vi "WPS_comm.vi"(0 "Path to Batch":string, 1 "Path to Exe":string, 2 "WPS IP:Port":string, 3 "Username":string, 4 "Password":string, 5 "Command":string) -> (14 "standard output":string, 15 "standard error":string, 16 "return code":i32, 19 "error out":errorcluster)   [LabVIEW 2016]
panel:
  out "Time (ms)":u32
  out "Complete command":string
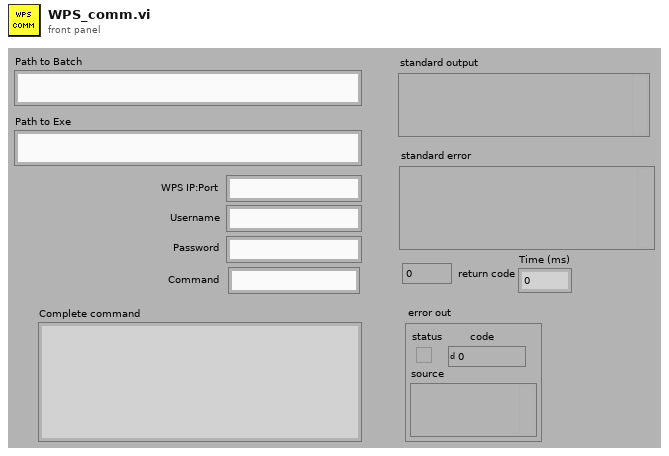
[diagram p1: front panel]
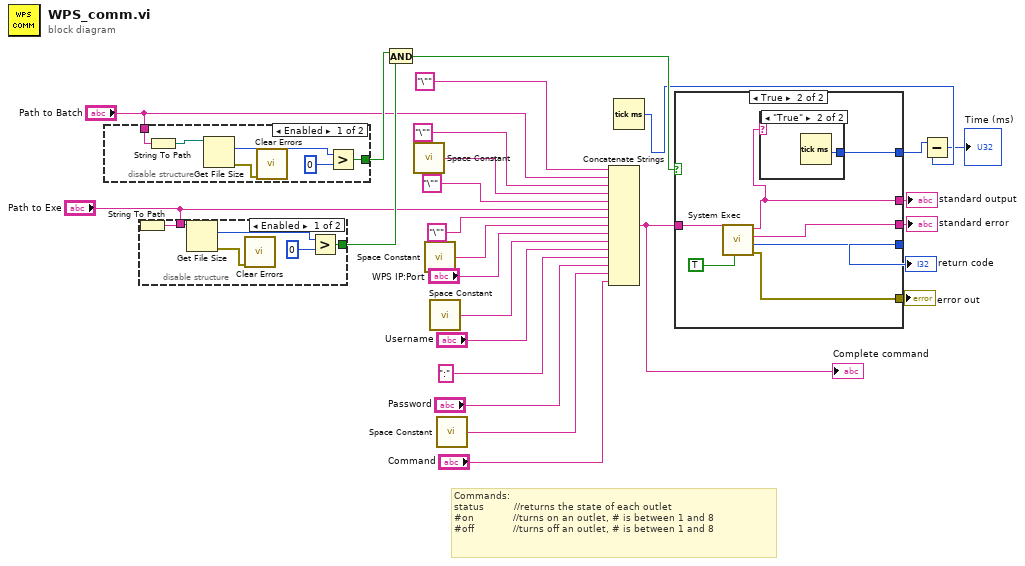
[diagram p0: block diagram]
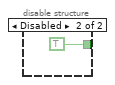
[diagram p2: hidden frame]
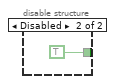
[diagram p3: hidden frame]
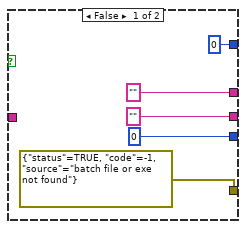
[diagram p4: hidden frame]
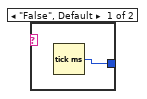
[diagram p5: hidden frame]
diagram:
  # "Commands:\nstatus          //returns the state of each outlet\n#on             //turns on an outlet, # is between 1 and 8\n#off             //turns off an outlet, # is between 1 and 8"
  n1 = disable-structure shown="Enabled" {
    disable-tunnel: [w30 TRUE] -> w7
    disable-tunnel: "Path to Batch" -> [w29 _]
    frame Enabled {
      n2 = String To Path(string=w29) -> (path=w28:path)
      n3 = Get File Size(file=w28) -> (size (in bytes)=w32:i64, 0:w27:errorcluster)  [unwired: 1 in, 1 out]
      n4 = call <vilib>:"Clear Errors.vi"("error in (no error)"=w27) -> ()  [unwired: 5 in, 2 out]
      n5 = Greater?(x=w32, y=i64 0) -> (0:w30:bool)
    }
    frame Disabled {
    }
  }
  n6 = disable-structure shown="Enabled" {
    disable-tunnel: [w37 TRUE] -> w6
    disable-tunnel: "Path to Exe" -> [w36 _]
    frame Enabled {
      n7 = String To Path(string=w36) -> (path=w35:path)
      n8 = Get File Size(file=w35) -> (size (in bytes)=w39:i64, 0:w34:errorcluster)  [unwired: 1 in, 1 out]
      n9 = call <vilib>:"Clear Errors.vi"("error in (no error)"=w34) -> ()  [unwired: 5 in, 2 out]
      n10 = Greater?(x=w39, y=i64 0) -> (0:w37:bool)
    }
    frame Disabled {
    }
  }
  n11 = And(x=w7, y=w6) -> (x .and. y?=w8:bool)
  n12 = call <vilib>:"Space Constant.vi"() -> ("String"=w11:string)
  n13 = call <vilib>:"Space Constant.vi"() -> ("String"=w16:string)
  n14 = call <vilib>:"Space Constant.vi"() -> ("String"=w15:string)
  n15 = call <vilib>:"Space Constant.vi"() -> ("String"=w14:string)
  n16 = Concatenate Strings("\"" ("string"), "Path to Batch", "\"" ("string"), w11, "\"" ("string"), "Path to Exe", "\"" ("string"), w16, "WPS IP:Port", w15, "Username", ":" ("string"), "Password", w14, "Command") -> (w19:string)
  "Complete command" <- w19
  n17 = Tick Count (ms)() -> (millisecond timer value=w2:u32)
  n18 = case shown="True" w8 {
    tunnel: ["" ("standard output") w47] -> w26
    tunnel: ["" ("standard error") w52] -> w25
    tunnel: [0 ("return code") w51] -> w24
    tunnel: [errorcluster {"status"=TRUE, "code"=-1, "source"="batch file or exe not found"} ("error out") w50] -> w23
    tunnel: w19 -> [_ w49]
    tunnel: [u32 0 ("millisecond timer value") w46] -> w3
    frame False {
    }
    frame True {
      n19 = call <vilib>:"System Exec.vi"("run minimized? (F)"=TRUE, "command line"=w49) -> ("error out"=w50:errorcluster, "return code"=w51:i32, "standard error"=w52:string, "standard output"=w47:string)  [unwired: 6 in]
      n20 = case shown="\"True\"" w47 {
        tunnel: [w53 w54] -> w46
        frame "False", Default {
          n21 = Tick Count (ms)() -> (millisecond timer value=w53:u32)
        }
        frame "True" {
          n22 = Tick Count (ms)() -> (millisecond timer value=w54:u32)
        }
      }
    }
  }
  "standard output" <- w26
  "standard error" <- w25
  "return code" <- w24
  "error out" <- w23
  n23 = Subtract(x=w3, y=w2) -> (x-y=→"Time (ms)":u32)
